vi "Odor_stimulation.vi"() -> ()   [LabVIEW 2009]
uses:
  <vilib>/Utility/file.llb/Read From Spreadsheet File (DBL).vi
panel:
  out "Duration of the Stimulation protocol (s)":i32
  out "Odor Channel (V)":dbl
  in  "Set frame size (ms) (minimum=2ms)":u32
  out "Odor Channel (V)":dbl[](graph)
  out "Length of the CSV file":i32
  out "Solvent Channel (V)":dbl[](graph)
  out "Solvent Channel (V)":dbl
  in  "Set Max Voltage (Combined flow of Channel 1 + Channel 2)\n(maximum=5V)":dbl=4.0
  in  "Stimulation START":bool
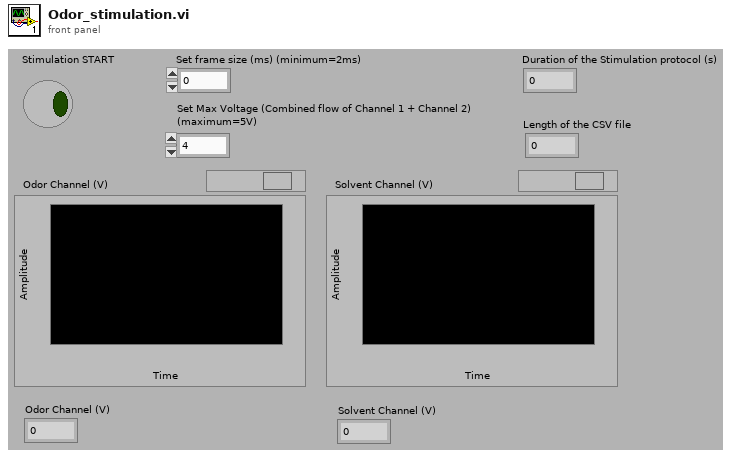
[diagram p1: front panel]
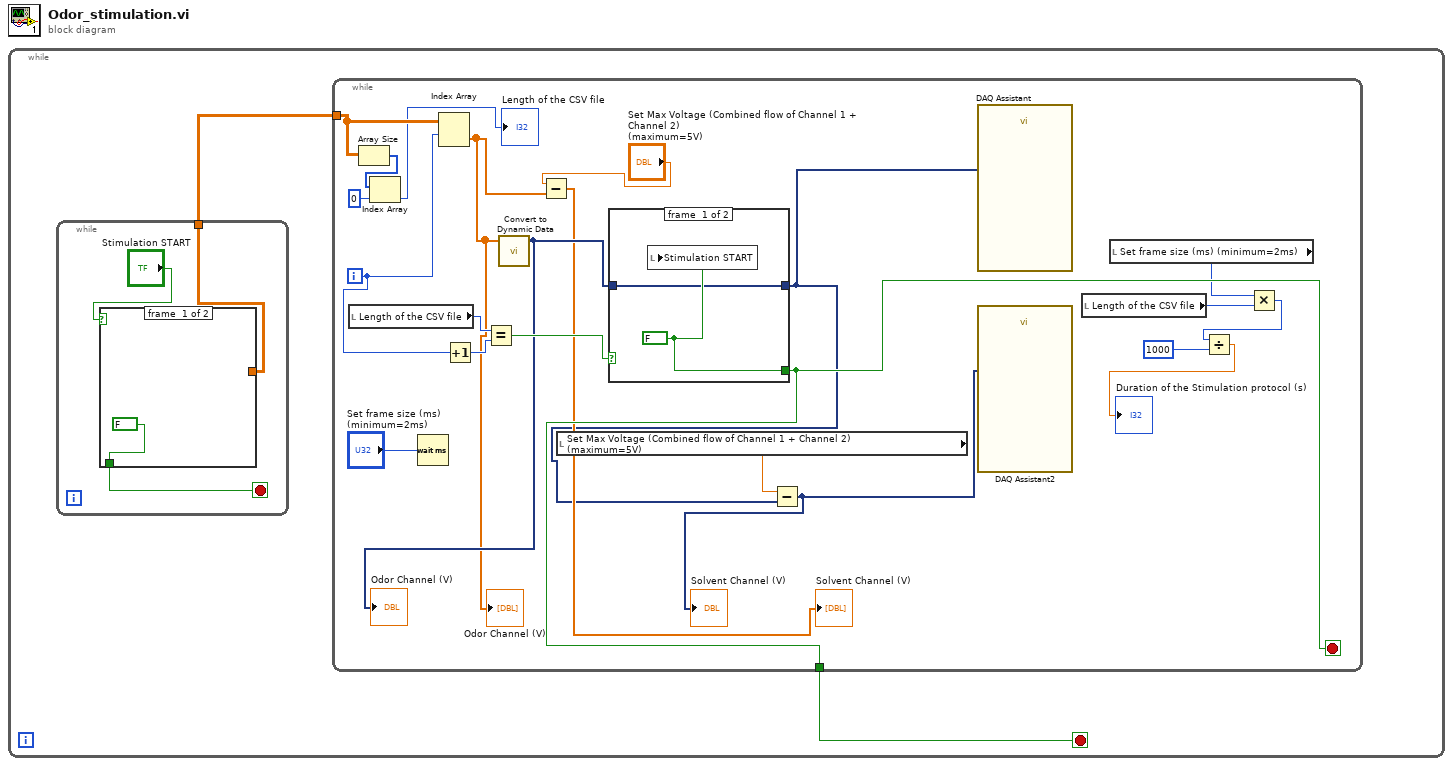
[diagram p0: block diagram]
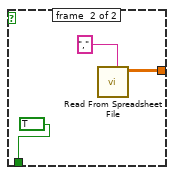
[diagram p2: hidden frame]
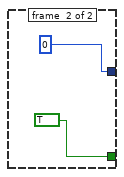
[diagram p3: hidden frame]
diagram:
  n1 = while {
    stop <- w1 stop-if-true
    n2 = while {
      tunnel: [w4] -> w2
      stop <- w5 stop-if-true
      n3 = case shown="True" "Stimulation START" {
        tunnel: [_ w7] -> w4
        tunnel: [FALSE TRUE] -> w5
        frame #0 {
        }
        frame #1 {
          n4 = call-poly <vilib>:"Read From Spreadsheet File.vi"("delimiter (\\t)"="," ("delimiter (\\t)")) -> ("all rows"=w7:dbl[][])  [unwired: 6 in, 4 out]
        }
      }
    }
    n5 = while {
      tunnel: w2 -> [w30]
      tunnel: [w23] -> w1
      i -> [w24]
      stop <- w23 stop-if-true
      n6 = local read "Length of the CSV file"() -> (w28:i32)
      n7 = Array Size(array=w30) -> (size(s)=w27:i32[])
      n8 = Index Array(array=w27, index=0) -> (element=→"Length of the CSV file":i32)
      n9 = Wait (ms)(milliseconds to wait="Set frame size (ms) (minimum=2ms)") -> ()  [unwired: 1 out]
      n10 = Index Array(array=w30, index (row)=w24) -> (element=w20:dbl[])  [unwired: 1 in]
      "Odor Channel (V)" <- w20
      n11 = Increment(x=w24) -> (x+1=w25:i32)
      n12 = Equal?(x=w28, y=w25) -> (x = y?=w29:bool)
      n13 = call "Convert to Dynamic Data"("Array"=w20) -> ("Dynamic Data Type"=w22:dynamicdata)  [unwired: 3 in]
      "Odor Channel (V)" <- w22
      n14 = Subtract(x="Set Max Voltage (Combined flow of Channel 1 + Channel 2)\n(maximum=5V)", y=w20) -> (x-y=→"Solvent Channel (V)":dbl[])
      n15 = local read "Set Max Voltage (Combined flow of Channel 1 + Channel 2)\n(maximum=5V)"() -> (w17:dbl)
      n16 = case shown="False" w29 {
        tunnel: [w33 TRUE] -> w23
        tunnel: w22 -> [w32 _]
        tunnel: [w32 0] -> w15
        frame #0 {
          w33 = FALSE
          n17 = local write "Stimulation START"(w33) -> ()
        }
        frame #1 {
        }
      }
      n18 = Subtract(x=w17, y=w15) -> (x-y=w16:dynamicdata)
      "Solvent Channel (V)" <- w16
      n19 = call "DAQ Assistant"("data"=w15) -> ()  [unwired: 17 in, 2 out]
      n20 = call "DAQ Assistant2"("data"=w16) -> ()  [unwired: 17 in, 2 out]
      n21 = local read "Length of the CSV file"() -> (w13:i32)
      n22 = local read "Set frame size (ms) (minimum=2ms)"() -> (w12:u32)
      n23 = Multiply(x=w12, y=w13) -> (x*y=w14:u32)
      n24 = Divide(x=w14, y=1000 ("index")) -> (x/y=→"Duration of the Stimulation protocol (s)":dbl)
    }
  }
